vi "reset_data.vi"(8 "error in (no error)":errorcluster, 11 "TTL_input in":refnum<class "TTL_input.lvclass">) -> (0 "error out":errorcluster, 3 "TTL_input out":refnum<class "TTL_input.lvclass">)   [LabVIEW 2013, in "TTL_input.lvclass"]
uses:
  TTL_input.lvclass
  TTL_input.lvclass/TTL_input.ctl
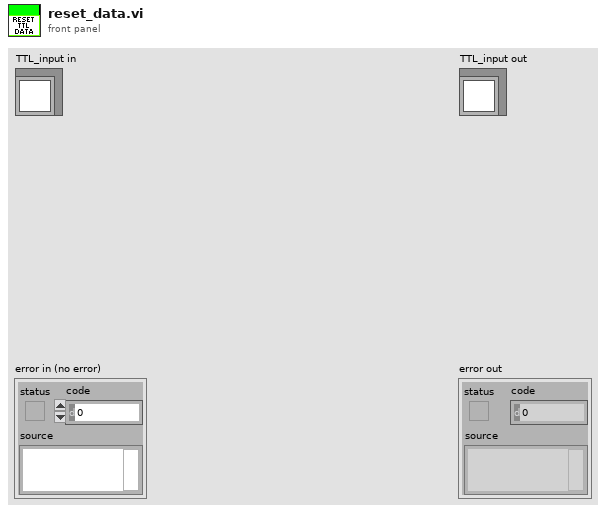
[diagram p1: front panel]
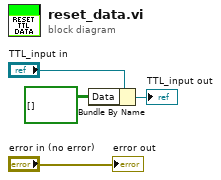
[diagram p0: block diagram]
diagram:
  n1 = Bundle By Name(cluster="TTL_input in", "Data"=bool[][] []) -> (→"TTL_input out":refnum<class "TTL_input.lvclass">)
  "error out" <- "error in (no error)"
